vi "InitWrapper.vi"(11 "DLLpath":path) -> (1 "MaxSpeed":dbl, 2 "MaxPower":dbl, 3 "Bed Size":cluster{"X":dbl, "Y":dbl})   [LabVIEW 2014]
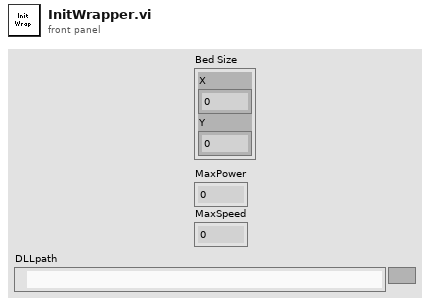
[diagram p1: front panel]
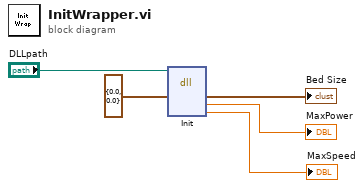
[diagram p0: block diagram]
diagram:
  n1 = dll-call lib="C:/Users/guss2/Desktop/DLLtest/MachineSimulator.dll" fn="Init"(path in="DLLpath", "BeamLoc"=cluster{"X":dbl, "Y":dbl} {"X"=0.0, "Y"=0.0} ("Bed Size")) -> ("BeamLoc"=→"Bed Size":cluster{"X":dbl, "Y":dbl}, "MaxPower"=→"MaxPower":dbl, "MaxSpeed"=→"MaxSpeed":dbl)  [unwired: 5 in, 2 out]
